vi "数据回读.vi"() -> ()   [LabVIEW 2013]
doc: "This example demonstrates how to acquire a continuous data."
panel:
  in  "单次回读采样点数":i64=1024
  in  "回放间隔ms":u32=200
  out "波形图":dbl[][](graph)
  out "数据":dbl[][](array[numeric])
  in  "停止按钮":bool
  out "使能通道名称":string
  in  "文件路径":path=path "C:/Users/Administrator/Desktop/Data.tdms"
  out "错误":errorcluster
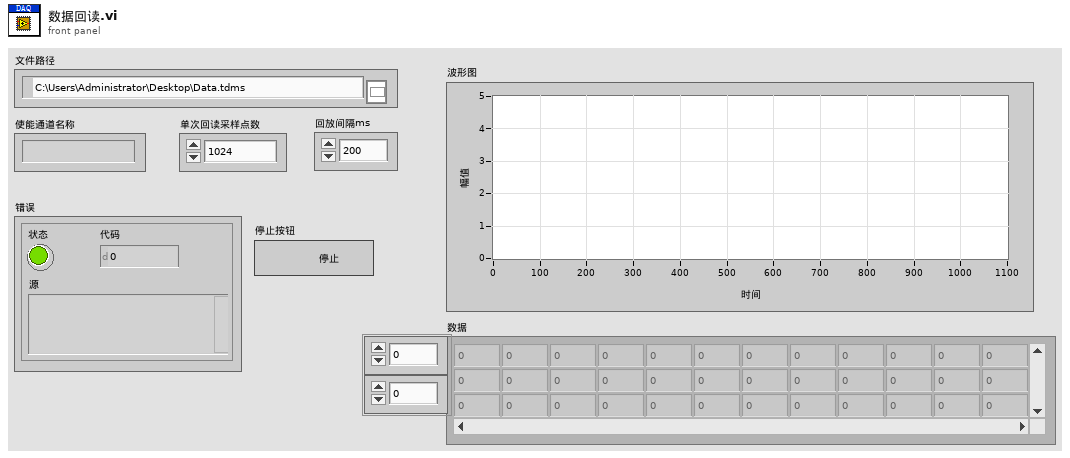
[diagram p1: front panel]
types:
  T1 = enum16{"open", "open or create", "create or replace", "create", "open (read-only)"}
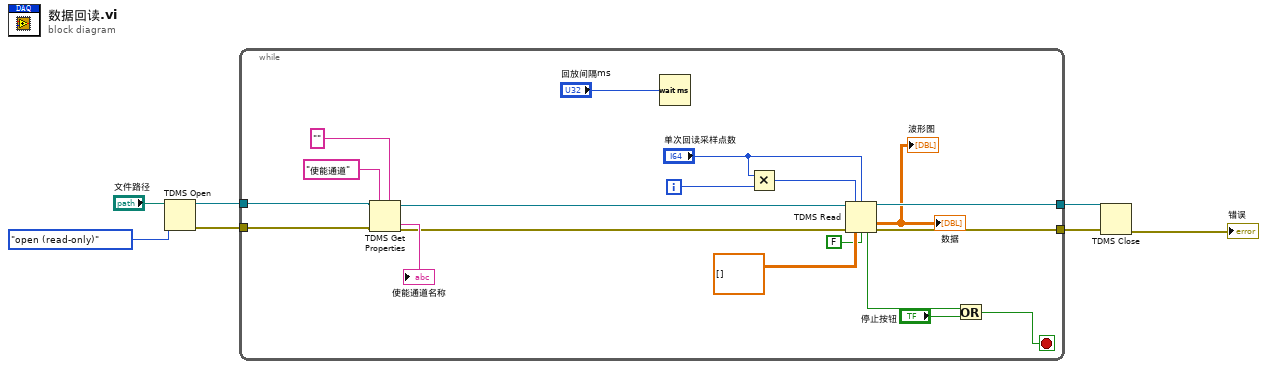
[diagram p0: block diagram]
diagram:
  n1 = TDMS Open(10:T1."open (read-only)" ("操作(0:open)"), 11:"文件路径") -> (0:w1:errorcluster, 3:w2:refnum<k34>)  [unwired: 5 in]
  n2 = while {
    tunnel: [w26] -> w5
    tunnel: [w25] -> w4
    tunnel: w2 -> [w24]
    tunnel: w1 -> [w23]
    i -> [w9]
    stop <- w10 stop-if-true
    n3 = TDMS Get Properties(5:"", 7:"使能通道", 8:w23, 11:w24) -> (0:w18:errorcluster, 3:w19:refnum<k34>, 4:→"使能通道名称":string)  [unwired: 2 in, 3 out]
    n4 = Wait (ms)(milliseconds to wait="回放间隔ms") -> ()  [unwired: 1 out]
    n5 = Multiply(x="单次回读采样点数", y=w9) -> (x*y=w11:i64)
    n6 = TDMS Read(0:w19, 1:w11, 2:"单次回读采样点数", 11:w18, 12:dbl[][] [], 13:FALSE ("按文件顺序返回通道？(F)")) -> (4:w26:refnum<k34>, 10:→"数据" →"波形图":dbl[][], 14:w15:bool, 15:w25:errorcluster)  [unwired: 2 in, 2 out]
    n7 = Or(x=w15, y="停止按钮") -> (x .or. y?=w10:bool)
  }
  n8 = TDMS Close(8:w4, 11:w5) -> (0:→"错误":errorcluster)  [unwired: 1 out]
